vi "rwfm_Start.vi"(8 "error in":errorcluster, 9 "IRQ Number (11)":i32=11, 10 "Sampling Info In":T2, 11 "Dynamic FPGA VI Reference":T1) -> (0 "error out":errorcluster, 2 "Sampling Info Out":T2, 3 "Dynamic FPGA VI Reference":T1)   [LabVIEW 2017, in "cRIOWfmLibMcsa.lvlib"]
doc: "This VI starts the FPGA and waits for the FPGA to send an interrupt signifying that it is ready to begin the acquisition. This VI can be called multiple times to restart a paused acquisition or to retrigger a finite acquisition. If the Start is called more than once, it throws a harmless warning (code 61003) saying the FPGA is already running."
uses:
  <vilib>/addons/InsightCM/Devices/Shared/Mcsa/cRIOWfmAcqMcsa/cRIOWfmLibMcsa.lvlib
  <vilib>/addons/InsightCM/Devices/Shared/Cms/cRIOWfmAcq/subVIs/RIO Wfm Cust Ctrls/rwfm_SamplingInfo.ctl
  <vilib>/addons/InsightCM/Devices/Shared/Mcsa/cRIOWfmAcqMcsa/controls/rwfm_DynamicFPGArefMCSA.ctl
  <vilib>/Utility/error.llb/Error Cluster From Error Code.vi
  <vilib>/rvi/interface/nirviMethod/nirviMethod.xnode
  <vilib>/addons/InsightCM/Devices/Shared/Cms/cRIOWfmAcq/cRIOWfmLib.lvlib
  <vilib>/rvi/interface/nirviMethod/StockFPGA_InlinedMethodWaitForSingleIRQ.vi
  <vilib>/FPGAPlugInAG/Dynamic/niLvFpga_WaitOnIrq_Dynamic.vi
  <vilib>/FPGAPlugInAG/Dynamic/niLvFpga_AcknowledgeIrq_Dynamic.vi
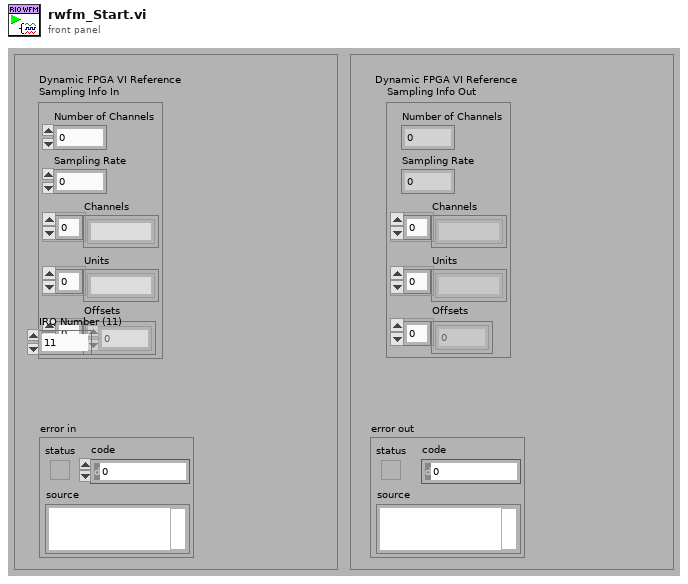
[diagram p1: front panel]
types:
  T1 = typedef "cRIOWfmLibMcsa.lvlib/rwfm_DynamicFPGArefMCSA.ctl" = refnum<k20>
  T2 = typedef "cRIOWfmLib.lvlib/rwfm_SamplingInfo.ctl" = cluster{"Number of Channels":i32, "Sampling Rate":dbl, "Channels":string[], "Units":string[], "Offsets":sgl[]}
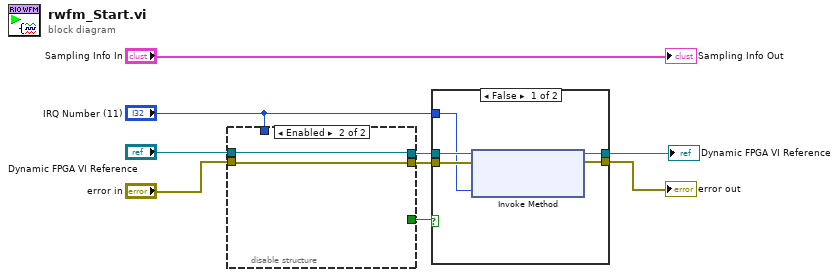
[diagram p0: block diagram]
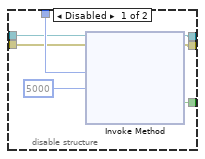
[diagram p2: hidden frame]
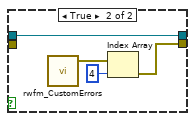
[diagram p3: hidden frame]
diagram:
  n1 = disable-structure shown="Enabled" {
    disable-tunnel: [w16 w18] -> w9
    disable-tunnel: [w15 w17] -> w8
    disable-tunnel: "IRQ Number (11)" -> [w14 _]
    disable-tunnel: [w12 _] -> w3
    disable-tunnel: "Dynamic FPGA VI Reference" -> [w11 w18]
    disable-tunnel: "error in" -> [w10 w17]
    frame Disabled {
      n2 = xnode "Invoke Method"("FPGA VI Reference In"=w11, "error in"=w10, "IRQ Number(s)"=w14, "Timeout (ms)"=5000) -> ("FPGA VI Reference Out"=w16:T1, "error out"=w15:errorcluster, "Timed Out"=w12:bool)  [unwired: 1 out]
    }
    frame Enabled {
    }
  }
  n3 = case shown="False" w3 {
    tunnel: w9 -> [w23 w27]
    tunnel: w8 -> [w22 _]
    tunnel: [w21 w27] -> w5
    tunnel: [w20 w24] -> w7
    tunnel: "IRQ Number (11)" -> [w19 _]
    frame False {
      n4 = xnode "Invoke Method"("FPGA VI Reference In"=w23, "error in"=w22, "IRQ Number(s)"=w19) -> ("FPGA VI Reference Out"=w21:T1, "error out"=w20:errorcluster)
    }
    frame True {
      n5 = call <vilib>:"rwfm_CustomErrors.vi"() -> ("Error Array"=w25:errorcluster[])  [unwired: 5 in]
      n6 = Index Array(array=w25, index=4) -> (element=w24:errorcluster)
    }
  }
  "error out" <- w7
  "Dynamic FPGA VI Reference" <- w5
  "Sampling Info Out" <- "Sampling Info In"
